vi "Set Processes.vi"(8 "Error In":errorcluster, 10 "Processes":T1, 11 "Dashboard In":refnum<class "Dashboard.lvclass">) -> (0 "Error Out":errorcluster, 3 "Dashboard Out":refnum<class "Dashboard.lvclass">)   [LabVIEW 2021, in "Dashboard.lvclass"]
uses:
  Dashboard.lvclass
  Private/Controls/Processes.ctl
  Display Manager/Display Manager.lvclass
  Audio Analyzer/Audio Analyzer.lvclass
  Draw Frame/Draw Frame.lvclass
  Error Handling/Error Handling.lvclass
  Sequencer/Sequencer.lvclass
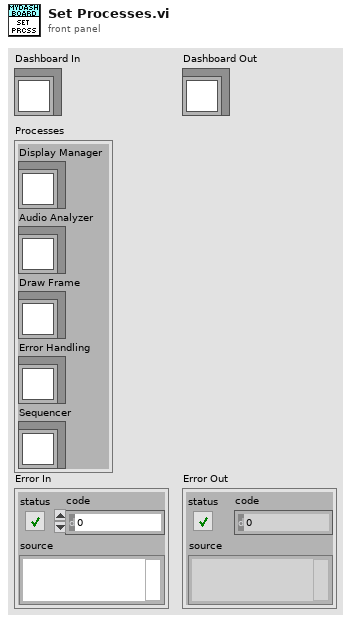
[diagram p1: front panel]
types:
  T1 = typedef "Dashboard.lvclass/Processes.ctl" = cluster{"Display Manager":refnum<class "Display Manager.lvclass">, "Audio Analyzer":refnum<class "Audio Analyzer.lvclass">, "Draw Frame":refnum<class "Draw Frame.lvclass">, "Error Handling":refnum<class "Error Handling.lvclass">, "Sequencer":refnum<class "Sequencer.lvclass">}
  T2 = typedef "Dashboard.lvclass/Data.ctl" = cluster{"Central Message Handler":refnum<class "Central Message Handler.lvclass">, "Display":refnum<class "Display.lvclass">, "FPGA Reference":T3, "Open Weather Session":refnum<class "Open Weather Session.lvclass">, "Processes":T1}
  T3 = typedef "Dashboard.lvclass/FPGA Reference.ctl" = refnum<k20>
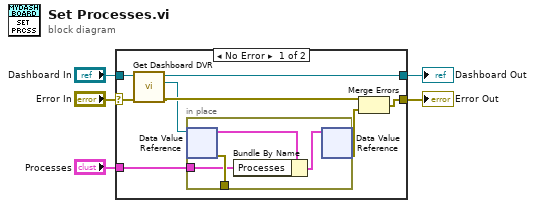
[diagram p0: block diagram]
diagram:
  n1 = case shown="No Error" "Error In" {
    selector: "Error In" -> [w9 w18]
    tunnel: [w12 w18] -> w2
    tunnel: [w8 w19] -> w5
    tunnel: "Dashboard In" -> [w10 w19]
    tunnel: "Processes" -> [w11 _]
    frame No Error {
      n2 = call "Get Dashboard DVR.vi"("Error In"=w9, "Dashboard In"=w10) -> ("Error Out"=w7:errorcluster, "DVR"=w6:refnum<data-value>, "Dashboard Out"=w8:refnum<class "Dashboard.lvclass">)  [unwired: 7 in]
      n3 = in-place {
        in-place-border: [w17] -> _
        in-place-border: w11 -> [w14]
        n4 = in-place-dvr #1(w6) -> (w16:T2, w17:errorcluster)
        n5 = Bundle By Name(cluster=w16, "Processes"=w14) -> (w15:T2)
        n6 = in-place-dvr #1(w15) -> (w13:errorcluster)  [unwired: 1 out]
      }
      n7 = Merge Errors(w7, w13) -> (w12:errorcluster)
    }
    frame Error {
    }
  }
  "Dashboard Out" <- w5
  "Error Out" <- w2
